vi "UI_Loading_Unit.vi"() -> ()   [LabVIEW 2014]
panel:
  out "DATA":T1
  in  "退出":bool
  # "加载单元监测参数"
  # "报警信息"
  # "KN"
  # "KN"
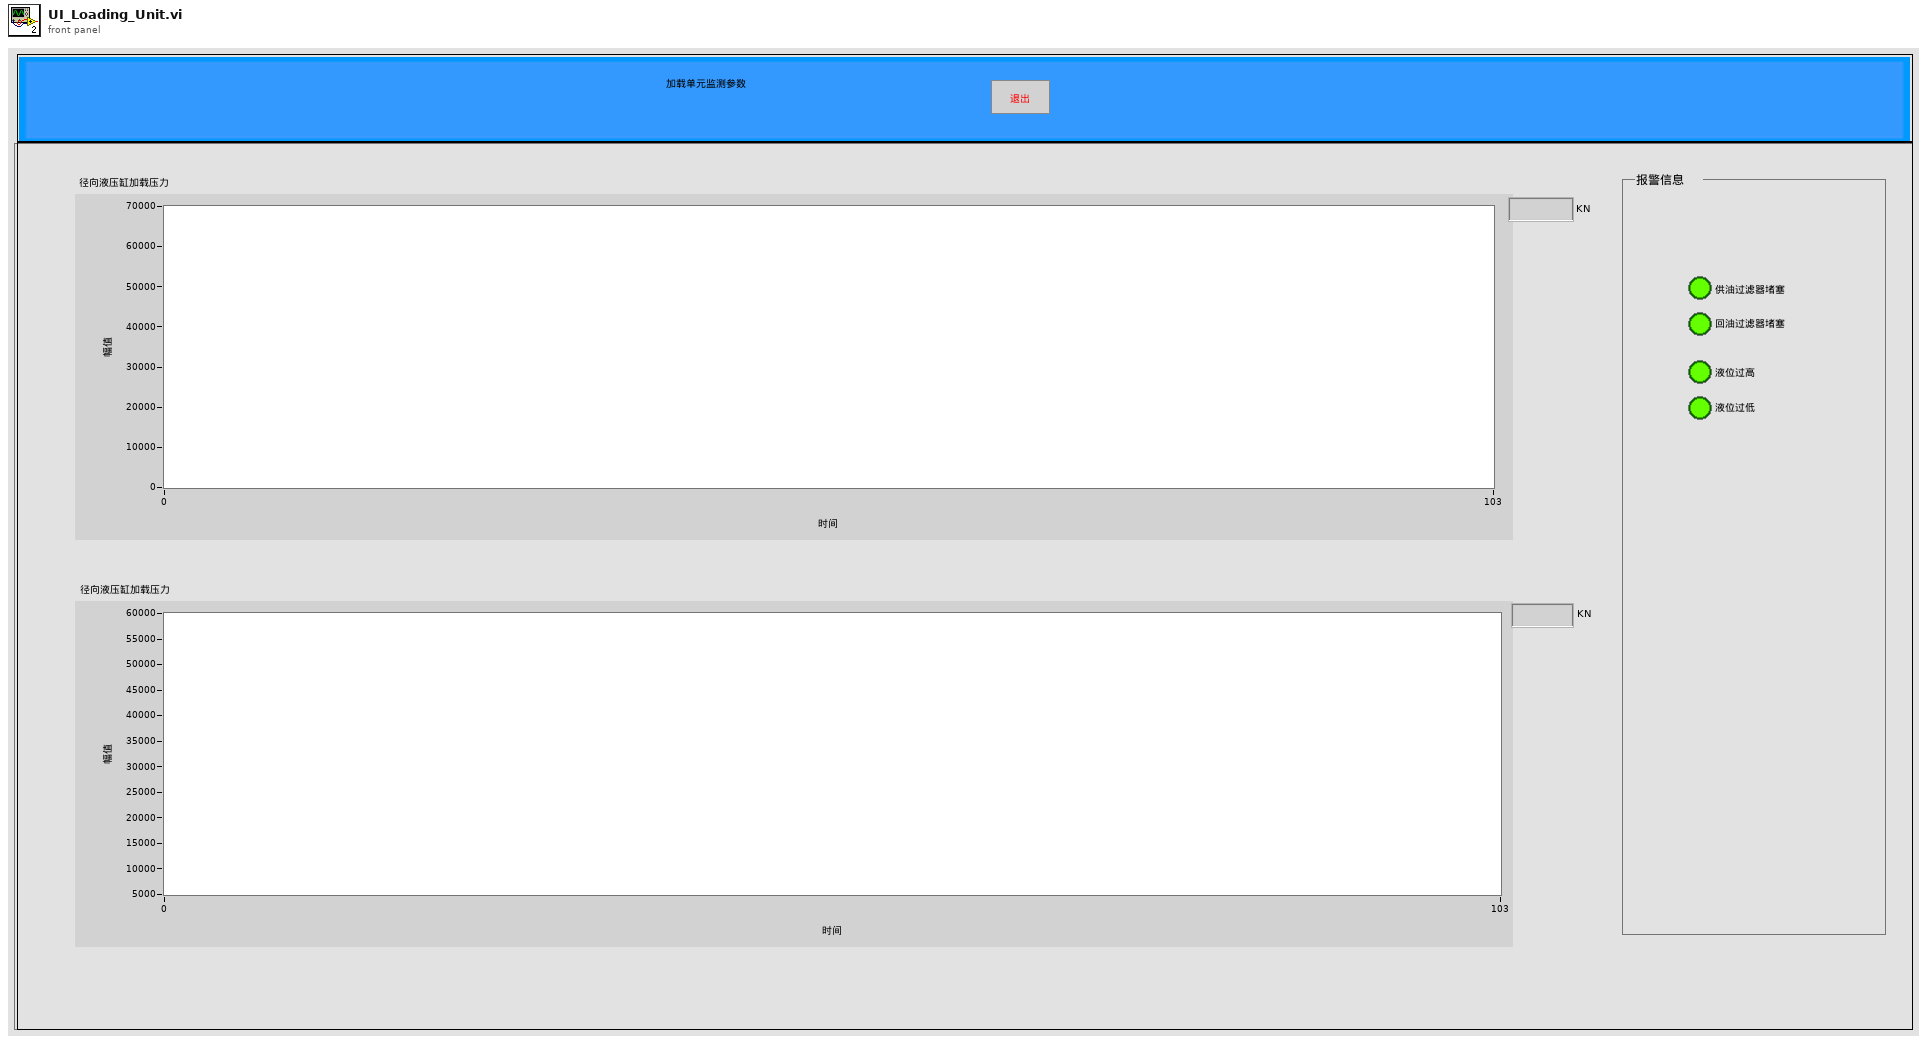
[diagram p1: front panel]
types:
  T1 = cluster{"径向液压缸加载压力":u16, "轴向液压缸加载压力":u16, "报警信息":cluster{"加载单元供油过滤器堵塞":bool, "加载单元回油过滤器堵塞":bool, "加载单元液位过高":bool, "加载单元单元液位过低":bool}}
  T2 = cluster{"径向油缸加载压力":u16, "轴向油缸加载压力":u16, "油箱1油液温度":u16, "润滑油温度":u16, "油箱2油液温度":u16, "试验轴承供油压力":u16, "试验轴承供油流量":u16, "陪试轴承供油流量":u16, "陪试轴承供油压力":u16, "陪试轴承供油温度":u16, "液压子系统状态字":cluster{"加载单元":cluster{"供油过滤器堵塞报警":bool, "回油过滤器堵塞报警":bool, "液位过高报警":bool, "液位过低报警":bool}, "试验轴承单元":cluster{"加热装置异常报警":bool, "油箱1液位过高报警":bool, "油箱1液位过低报警":bool, "油箱2液位过高报警":bool, "油箱2液位过低报警":bool, "供油过滤器堵塞报警":bool, "循环回路过滤器堵塞报警":bool, "回油过滤器堵塞报警":bool}, "陪试轴承单元":cluster{"供油过滤器1堵塞报警":bool, "供油过滤器2堵塞报警":bool, "回油过滤器堵塞报警":bool, "油箱液位过高报警":bool, "油箱液位过低报警":bool}}}
  T3 = cluster{"供油过滤器1堵塞报警":bool, "供油过滤器2堵塞报警":bool, "回油过滤器堵塞报警":bool, "油箱液位过高报警":bool, "油箱液位过低报警":bool}
  T4 = cluster{"供油过滤器堵塞报警":bool, "回油过滤器堵塞报警":bool, "液位过高报警":bool, "液位过低报警":bool}
  T5 = cluster{"径向油缸加载压力":u16, "轴向油缸加载压力":u16, "加载单元":cluster{"供油过滤器堵塞报警":bool, "回油过滤器堵塞报警":bool, "液位过高报警":bool, "液位过低报警":bool}}
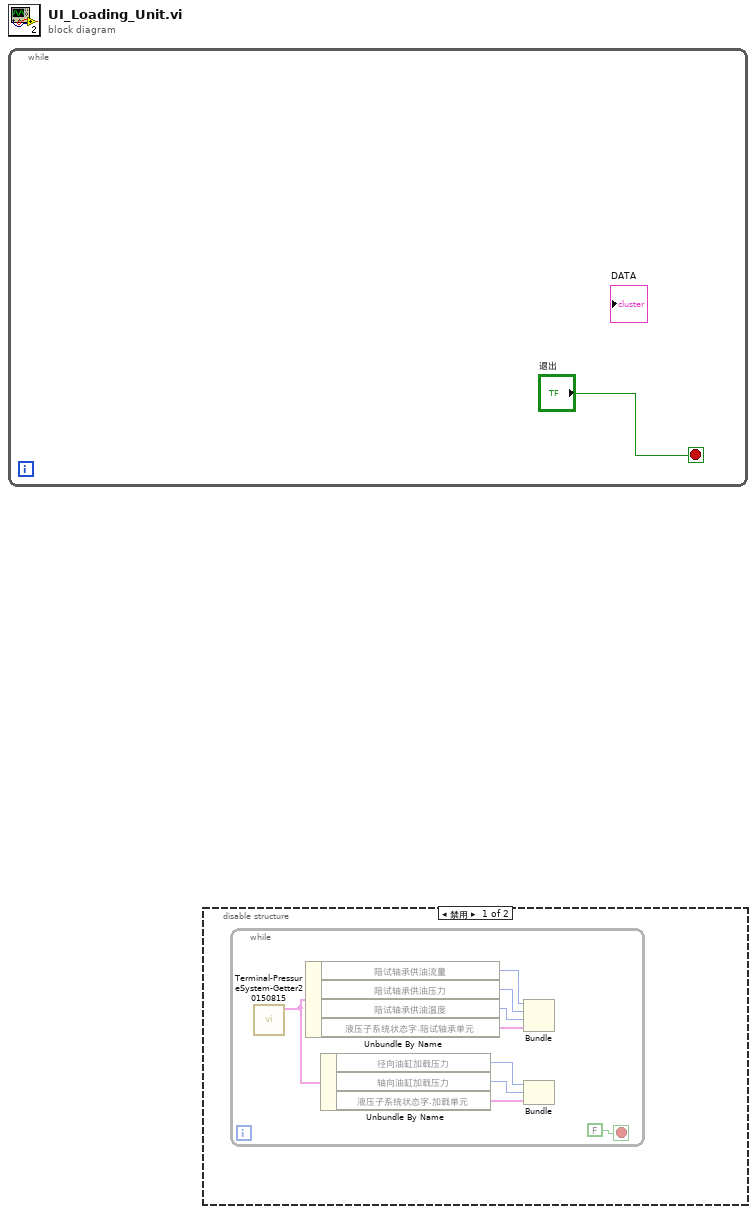
[diagram p0: block diagram]
diagram:
  n1 = while {
    stop <- "退出" stop-if-true
  }
  n2 = disable-structure shown="禁用" {
    frame Disabled {
      n3 = while {
        stop <- FALSE stop-if-true
        n4 = call "Terminal-PressureSystem-Getter20150815.vi"() -> ("设备信息"=w6:T2)  [unwired: 9 in, 2 out]
        n5 = Unbundle By Name(w6) -> ("陪试轴承供油流量"=w9:u16, "陪试轴承供油压力"=w8:u16, "陪试轴承供油温度"=w7:u16, "液压子系统状态字.陪试轴承单元"=w10:T3)
        n6 = Unbundle By Name(w6) -> ("径向油缸加载压力"=w5:u16, "轴向油缸加载压力"=w4:u16, "液压子系统状态字.加载单元"=w3:T4)
        n7 = Bundle("陪试轴承供油流量"=w9, "陪试轴承供油压力"=w8, "陪试轴承供油温度"=w7, "陪试轴承单元"=w10) -> ()  [unwired: 1 in, 1 out]
        n8 = Bundle("径向油缸加载压力"=w5, "轴向油缸加载压力"=w4, "加载单元"=w3) -> (w2:T5)  [unwired: 1 in]
      }
    }
    frame Enabled {
    }
  }
